vi "final-Vi.vi"() -> ()   [LabVIEW 2018]
uses:
  <vilib>/Analysis/3filter.llb/Filter Passband Type.ctl
  <vilib>/Utility/file.llb/Read Delimited Spreadsheet (string).vi
  <vilib>/Analysis/3filter.llb/Butterworth Filter (DBL).vi
  <vilib>/Utility/file.llb/Read Delimited Spreadsheet (DBL).vi
  <vilib>/Analysis/NI_AAL_SigProc.lvlib
  <vilib>/Analysis/NI_AALBase.lvlib
  <vilib>/Analysis/NI_AALPro.lvlib
panel:
  out "平均心跳(BPM)":dbl
  out "?":bool
  out "RMSSD(ms)":dbl
  out "Mean R-R interval":dbl
  out "心跳(BPM)":dbl
  in  "sampling freq: fs":dbl=250.0 format="%0.2f"
  in  "order":i32=8
  in  "filter type":T1=enum."Bandpass"
  out "Power Spectrum":T2(graph)
  out "我們計算的RR":cluster{dbl[], dbl[]}(graph)
  in  "RR threshold":dbl=231.0 format="%0.2f"
  in  "filter higher  stop freq":dbl(slide)=30.96161616161616 scale=0.4..50.0
  out "RMSSD(ms)":dbl
  out "Mean R-R interval":dbl
  out "RR":cluster{dbl[], dbl[]}(graph)
  in  "filter lower stop freq":dbl(slide)=5.05050505050505 scale=0.0..10.0
  out "Band filter":cluster{dbl[], "Filtered X":dbl[]}[](graph)
  out "Origin ECG":cluster{dbl[], i32[]}(graph)
  # "RMSSD越大，\n表示副交感神經作用越強"
  # "一般正常心跳約為50~100下/分鐘"
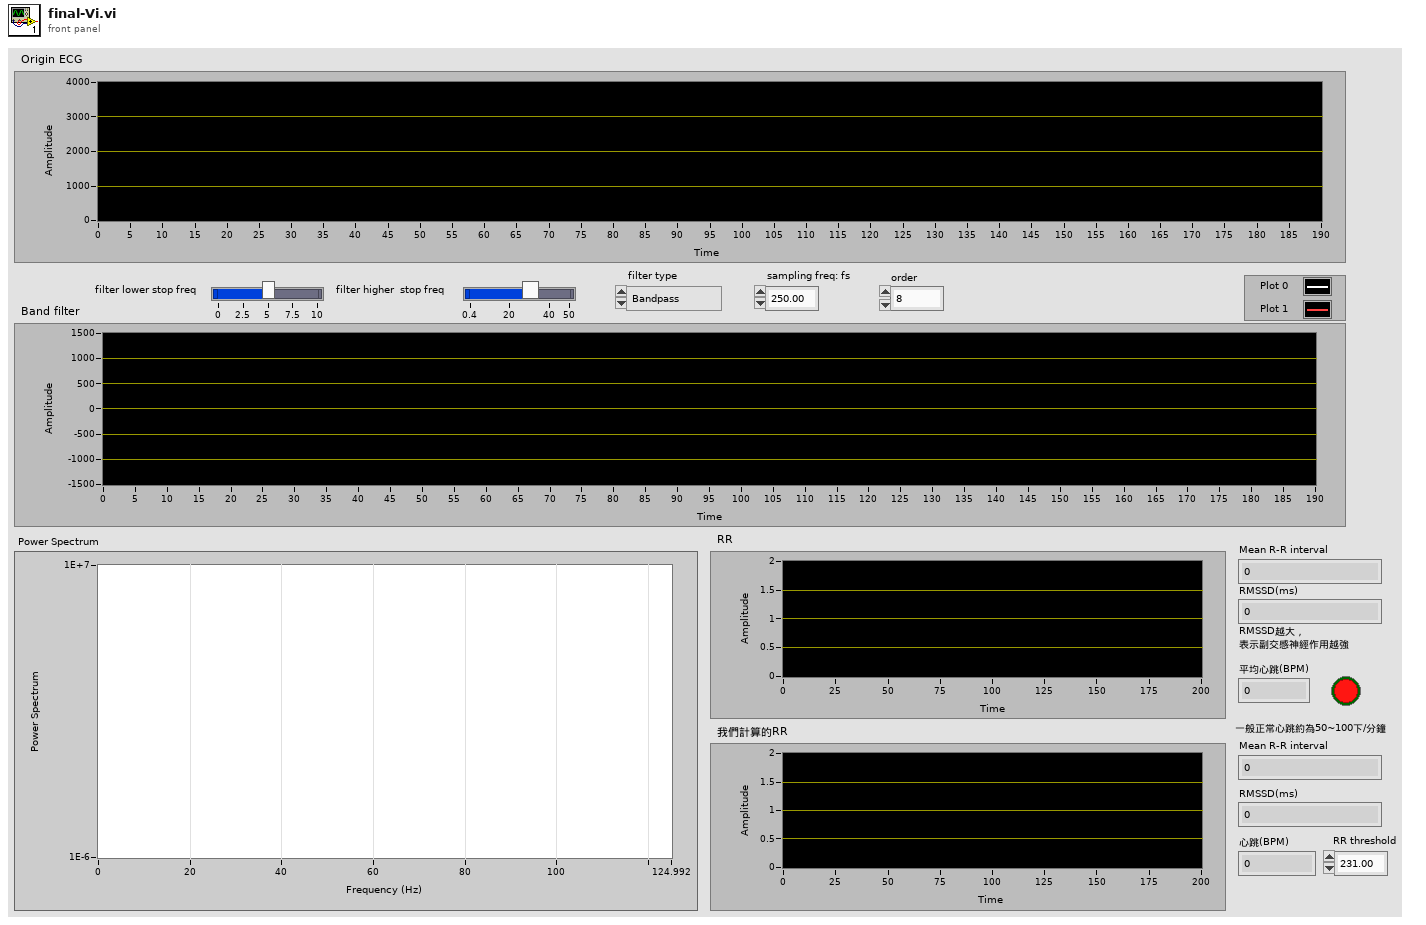
[diagram p1: front panel]
types:
  T1 = typedef "NI_AALBase.lvlib/Filter Passband Type.ctl" = enum32{"Lowpass", "Highpass", "Bandpass", "Bandstop"}
  T2 = cluster{"df":dbl, dbl, "Power Spectrum (V^2 rms)":dbl[]}
  T3 = cluster{dbl, "df":dbl, "Power Spectrum (V^2 rms)":dbl[]}
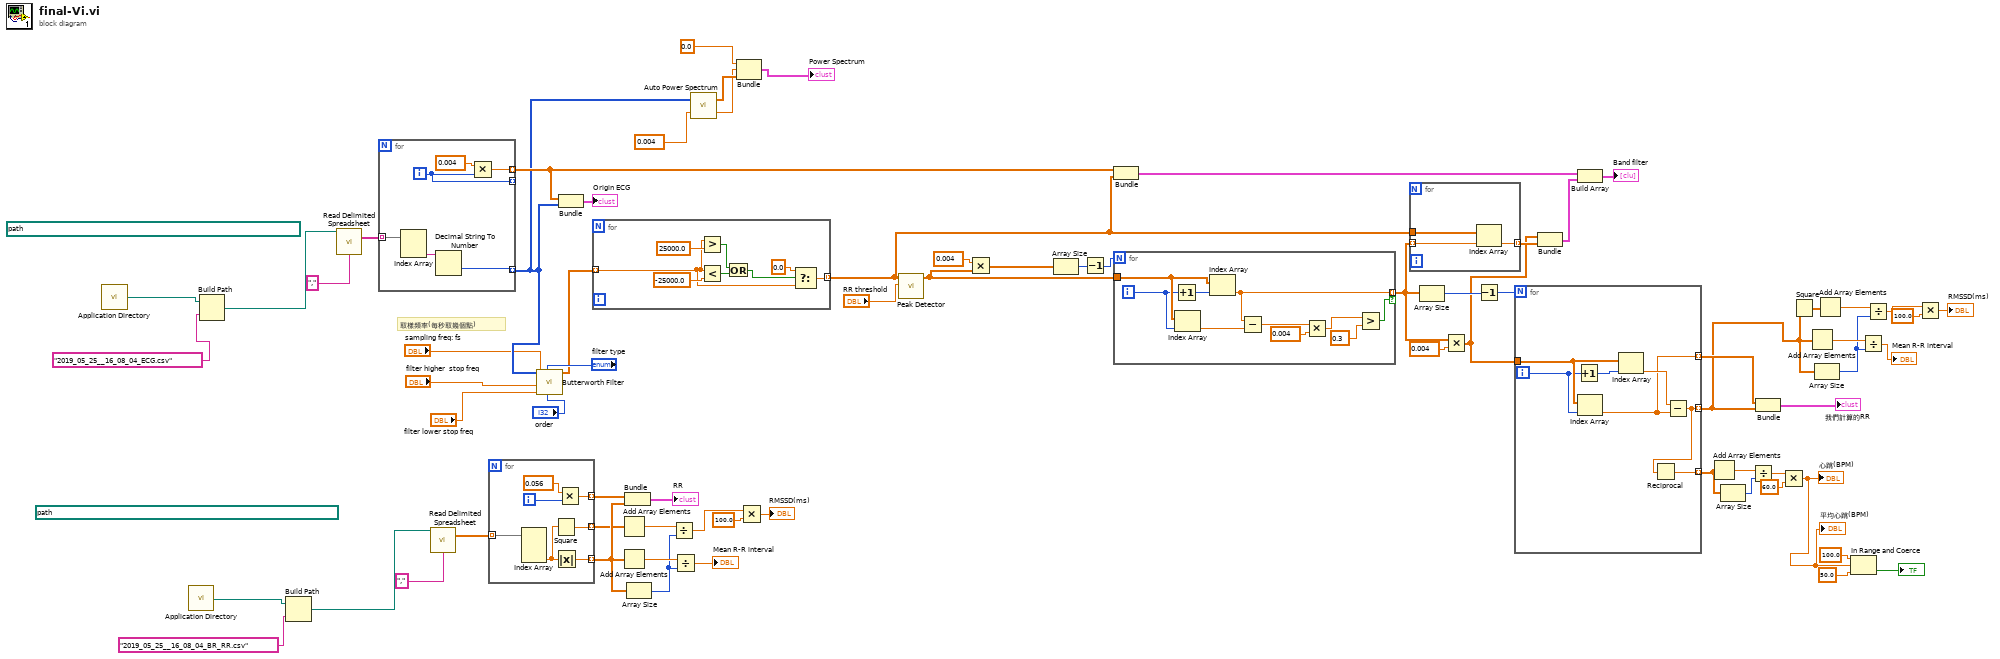
[diagram p0: block diagram]
diagram:
  (unwired) path "D:/Documents/生醫儀表/data/2019_05_25__14_12_20_BR_RR.csv" ("file path (dialog if empty)")
  (unwired) path "D:/Documents/生醫儀表/data/2019_05_25__14_12_20_ECG.csv" ("file path (dialog if empty)")
  # "取樣頻率(每秒取幾個點)"
  n1 = call <vilib>:"Application Directory.vi"() -> ("Application Directory"=w4:path)
  n2 = call <vilib>:"Application Directory.vi"() -> ("Application Directory"=w3:path)
  n3 = Build Path(base path=w4, name or relative path="2019_05_25__16_08_04_ECG.csv" ("file path (dialog if empty)")) -> (appended path=w5:path)
  n4 = Build Path(base path=w3, name or relative path="2019_05_25__16_08_04_BR_RR.csv" ("file path (dialog if empty)")) -> (appended path=w1:path)
  n5 = call-poly <vilib>:"Read Delimited Spreadsheet.vi"("file path (dialog if empty)"=w5, "delimiter (\\t)"="," ("delimiter (\\t)")) -> ("all rows"=w70:string[][])  [unwired: 8 in, 5 out]
  n6 = for {
    tunnel: w70 -> [w77] mode=indexing
    tunnel: [w72] -> w28 mode=indexing
    tunnel: [w76] -> w37 mode=indexing
    tunnel: [w74] -> _ mode=indexing
    i -> [w74]
    n7 = Index Array(array=w77) -> (element #2=w75:string)  [unwired: 2 in, 1 out]
    n8 = Decimal String To Number(string=w75) -> (number=w72:i32)  [unwired: 2 in, 1 out]
    n9 = Multiply(x=0.004 ("y"), y=w74) -> (x*y=w76:dbl)
  }
  n10 = call-poly <vilib>:"Read Delimited Spreadsheet.vi"("file path (dialog if empty)"=w1, "delimiter (\\t)"="," ("delimiter (\\t)")) -> ("all rows"=w69:dbl[][])  [unwired: 8 in, 5 out]
  n11 = for {
    tunnel: w69 -> [w84] mode=indexing
    tunnel: [w81] -> w68 mode=indexing
    tunnel: [w80] -> w64 mode=indexing
    tunnel: [w78] -> w63 mode=indexing
    i -> [w83]
    n12 = Index Array(array=w84) -> (element #3=w79:dbl)  [unwired: 3 in, 2 out]
    n13 = Square(x=w79) -> (x^2=w78:dbl)
    n14 = Absolute Value(x=w79) -> (abs(x)=w80:dbl)
    n15 = Multiply(x=0.056 ("y"), y=w83) -> (x*y=w81:dbl)
  }
  n16 = call-poly <vilib>:"Butterworth Filter.vi"("order"="order", "filter type"="filter type", "low cutoff freq: fl"="filter lower stop freq", "high cutoff freq: fh"="filter higher  stop freq", "sampling freq: fs"="sampling freq: fs", "X"=w28) -> ("Filtered X"=w31:dbl[])  [unwired: 2 in, 1 out]
  n17 = Bundle(w37, w28) -> (→"Origin ECG":cluster{dbl[], i32[]})  [unwired: 1 in]
  n18 = for {
    tunnel: w31 -> [w86] mode=indexing
    tunnel: [w85] -> w44 mode=indexing
    n19 = Greater?(x=w86, y=25000.0) -> (0:w90:bool)
    n20 = Less?(x=w86, y=-25000.0) -> (x < y?=w89:bool)
    n21 = Or(x=w90, y=w89) -> (x .or. y?=w88:bool)
    n22 = Select(t=0.0, s=w88, f=w86) -> (s? t:f=w85:dbl)
  }
  n23 = Add Array Elements(numeric array=w63) -> (sum=w62:dbl)
  n24 = Add Array Elements(numeric array=w64) -> (sum=w65:dbl)
  n25 = Bundle(w68, w64) -> (→"RR":cluster{dbl[], dbl[]})  [unwired: 1 in]
  n26 = Array Size(array=w64) -> (size(s)=w61:i32)
  n27 = Divide(x=w62, y=w61) -> (x/y=w60:dbl)
  n28 = Divide(x=w65, y=w61) -> (x/y=→"Mean R-R interval":dbl)
  n29 = call <vilib>:"Auto Power Spectrum.vi"("dt"=0.004, "Signal (V)"=w28) -> ("df"=w27:dbl, "Power Spectrum (V^2 rms)"=w30:dbl[])
  n30 = Bundle(0.0, "df"=w27, "Power Spectrum (V^2 rms)"=w30) -> (→"Power Spectrum":T3)  [unwired: 1 in]
  n31 = Multiply(x=w60, y=100.0) -> (x*y=→"RMSSD(ms)":dbl)
  n32 = call <vilib>:"Peak Detector.vi"("threshold"="RR threshold", "X"=w44) -> ("Locations"=w39:dbl[])  [unwired: 5 in, 4 out]
  n33 = Multiply(x=0.004 ("y"), y=w39) -> (x*y=w48:dbl[])
  n34 = Array Size(array=w48) -> (size(s)=w49:i32)
  n35 = Decrement(x=w49) -> (x-1=w42:i32)
  n36 = Bundle(w37, w44) -> (w53:cluster{dbl[], dbl[]})  [unwired: 1 in]
  n37 = for {
    N: w42 -> [_]
    tunnel: w39 -> [w102]
    tunnel: [w94] -> w41 mode=indexing if=w96
    i -> [w101]
    n38 = Increment(x=w101) -> (x+1=w100:i32)
    n39 = Index Array(array=w102, index=w101) -> (element=w95:dbl)
    n40 = Index Array(array=w102, index=w100) -> (element=w94:dbl)
    n41 = Subtract(x=w94, y=w95) -> (x-y=w98:dbl)
    n42 = Multiply(x=w98, y=0.004) -> (x*y=w97:dbl)
    n43 = Greater?(x=w97, y=0.3) -> (0:w96:bool)
  }
  n44 = for {
    tunnel: w41 -> [w104] mode=indexing
    tunnel: w44 -> [w105]
    tunnel: [w103] -> w51 mode=indexing
    n45 = Index Array(array=w105, index=w104) -> (element=w103:dbl)
  }
  n46 = Array Size(array=w41) -> (size(s)=w46:i32)
  n47 = Multiply(x=w41, y=0.004) -> (x*y=w40:dbl[])
  n48 = Decrement(x=w46) -> (x-1=w45:i32)
  n49 = for {
    N: w45 -> [_]
    tunnel: w40 -> [w112]
    tunnel: [w107] -> w16 mode=indexing
    tunnel: [w108] -> w38 mode=indexing
    tunnel: [w106] -> w23 mode=indexing
    i -> [w109]
    n50 = Increment(x=w109) -> (x+1=w111:i32)
    n51 = Index Array(array=w112, index=w109) -> (element=w108:dbl)
    n52 = Index Array(array=w112, index=w111) -> (element=w110:dbl)
    n53 = Subtract(x=w110, y=w108) -> (x-y=w107:dbl)
    n54 = Reciprocal(x=w107) -> (1/x=w106:dbl)
  }
  n55 = Bundle(w40, w51) -> (w50:cluster{dbl[], dbl[]})  [unwired: 1 in]
  n56 = Build Array(w53, w50) -> (→"Band filter":cluster{dbl[], dbl[]}[])
  n57 = Add Array Elements(numeric array=w23) -> (sum=w24:dbl)
  n58 = Array Size(array=w23) -> (size(s)=w22:i32)
  n59 = Divide(x=w24, y=w22) -> (x/y=w21:dbl)
  n60 = Bundle(w38, w16) -> (→"我們計算的RR":cluster{dbl[], dbl[]})  [unwired: 1 in]
  n61 = Multiply(x=w21, y=60.0) -> (x*y=w7:dbl)
  "心跳(BPM)" <- w7
  "平均心跳(BPM)" <- w7
  n62 = Square(x=w16) -> (x^2=w15:dbl[])
  n63 = Add Array Elements(numeric array=w16) -> (sum=w19:dbl)
  n64 = Array Size(array=w16) -> (size(s)=w17:i32)
  n65 = Add Array Elements(numeric array=w15) -> (sum=w18:dbl)
  n66 = In Range and Coerce(upper limit=100.0, x=w7, lower limit=50.0) -> (In Range?=→"?":bool)  [unwired: 1 out]
  n67 = Divide(x=w19, y=w17) -> (x/y=→"Mean R-R interval":dbl)
  n68 = Divide(x=w18, y=w17) -> (x/y=w12:dbl)
  n69 = Multiply(x=w12, y=100.0) -> (x*y=→"RMSSD(ms)":dbl)
